vi "00_MOD_Instrument_IO.vi"(8 "error in":errorcluster, 11 "Main Config File Refnum":T2) -> (0 "error out":errorcluster)   [LabVIEW 2018]
doc: "Instrument IO Module main VI. This is the critical Timed loop of the NGTS system. \n\nIt configures DAQmx tasks and channels for PXI, SCXI, and FieldPoint banks for cFP (and future other) instrument buses/cards/modules/banks. The configurations are loaded from tab delimited text files that contain the Tags, Addresses, scaling, polarity, IO type, and other physical IO based Tags. These files are normally located in the \\Config_Files subdirectory. Data IO. Other than an initial channel location .iak file for cFP, all Tags are defined programmatically, without NI-MAX.\n\nIt runs the IO tasks at a nominal 100 mS loop rate. This is adjustable. Data is sent to/from other parts of the system using a Smart VIGlobal, or optionally simple VIGlobals, or RT FIFOs.\n\n2007_11 Mike Ashe\nmichael.ashe@imaginatics.net\nCell: 860-961-0876"
uses:
  <vilib>/Platform/TimedLoop/XDataNode/wakeup.ctl
  <vilib>/Platform/TimedLoop/XDataNode/XDNodeRunTimeDep.lvlib
  <vilib>/Platform/TimedLoop/XDataNode/nitl_modes.ctl
  <vilib>/Platform/TimedLoop/XDataNode/timing_clust.ctl
  <vilib>/Platform/TimedLoop/XDataNode/XDataNode.xnode
  <vilib>/Utility/config.llb/NI_LVConfig.lvlib
  Common/Controls/ENUM Get-Load Action.ctl
  <resource>/objmgr/daqmx.rc
  <vilib>/Utility/config.llb/Read Key (String).vi
  <vilib>/Utility/config.llb/Config Data RefNum.ctl
panel:
  out "x-y":u32
  in  "stop":bool
  out "Period":i64
  out "appended array":dbl[](array[numeric])
  out "error IO":errorcluster
  in  "Error Action":T1(radio)
  in  "Wait On Error?":bool
  in  "Error Wait(mS)":i32=1000
  out "AO Values":dbl[](array[numeric])
  out "Main Loop Period":cluster{i64, "Iteration Duration":i64}(graph)
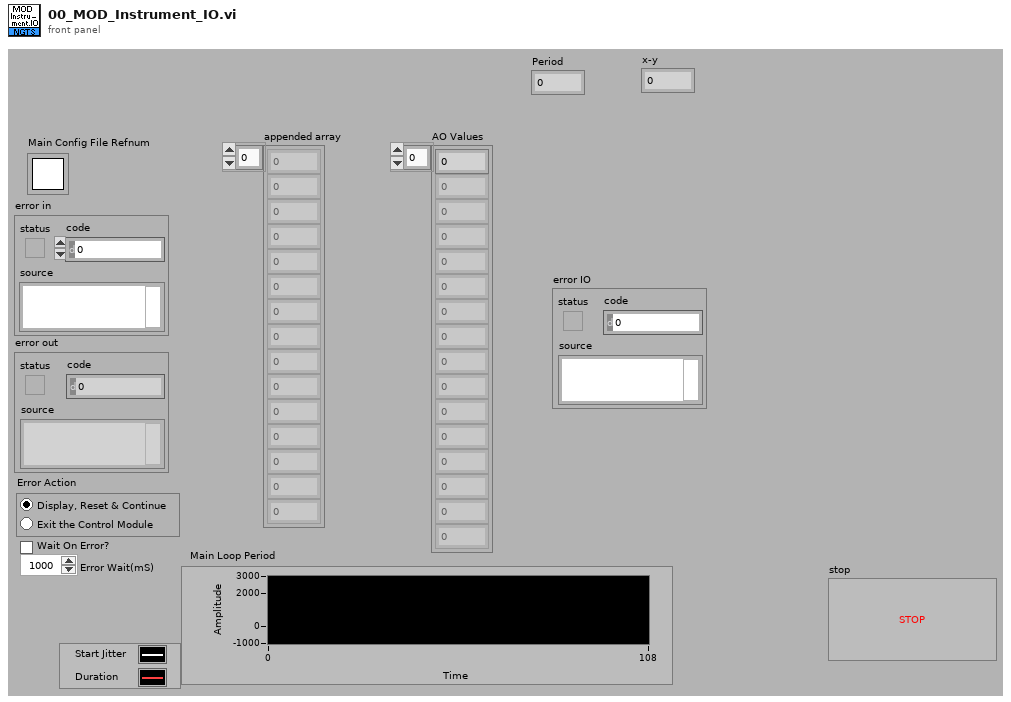
[diagram p1: front panel]
types:
  T1 = enum32{"Display, Reset & Continue", "Exit the Control Module"}
  T2 = typedef "NI_LVConfig.lvlib/Config Data RefNum.ctl" = refnum<k1>
  T3 = typedef "Instrument_IO Shift Variables.ctl" = cluster{"error":errorcluster, "AI_Tasks_State":T4, "AO_Tasks_State":T4, "RUN_PMT_AI":bool, "RUN_PMT_AO":bool, "RUN_PMT_DI":bool, "WDT Time Stamp 1":timestamp, "WDT Time Stamp 2":timestamp, "RT_TO":i32, "WDT_TO":dbl, "AO Tasks":refnum<k21>[], "DI Tasks":refnum<k21>[], "Tag Set Directory":path, "LogPath":path, "DI_Tasks_State":T4, "DO Tasks":refnum<k21>[], "RUN_PMT_DO":bool, "DO_Tasks_State":T4, "LogErrors?":bool, "System Type":string, "AI Sample Rate":dbl, "Timed Loop Rate":dbl, "AI Averaging On":bool, "Agilent Visa Resource":refnum<visa-resource-name>, "FEM Visa Resource":refnum<visa-resource-name>, "AI Tasks":refnum<k21>}
  T4 = typedef "MM_Module_Action.ctl" = enum16{"Idle", "Start", "Run", "Exit"}
  T5 = typedef "XDNodeRunTimeDep.lvlib/timing_clust.ctl" = cluster{"Expected End [f-1]":u64, "Actual End [f-1]":u64, "Finished Late? [f-1]":bool, "Expected End [i-1]":u64, "Actual End [i-1]":u64, "Finished Late? [i-1]":bool, "Expected Start [i]":u64, "Actual Start [i]":u64, "Expected Start [f]":u64, "Actual Start [f]":u64, "Source Name":string, "Structure Name":string, "Period":i64, "Deadline":i64, "Offset":i64, "Start":i64, "Priority":i32, "Timeout":i32, "Mode":T6, "Wakeup Reason":T7, "Error":errorcluster, "Source Type":string, "Secondary Source Type":string, "Global End Time":u64, "Global Start Time":u64, "Frame Duration":u64, "Iteration Duration":u64, "Assigned CPU":i32, "I/O Scan Engine Mode":u32}
  T6 = typedef "XDNodeRunTimeDep.lvlib/nitl_modes.ctl" = enum32{"No Change", "Process missed periods, maintain original phase", "Discard missed periods, maintain original phase", "Process missed periods, ignore original phase", "Discard missed periods, ignore original phase"}
  T7 = typedef "XDNodeRunTimeDep.lvlib/wakeup.ctl" = enum32{"Normal", "Aborted", "Asynchronous wakeup", "Timing source error", "Timed loop error", "Timeout"}
  T8 = typedef "ENUM Get-Load Action.ctl" = enum16{"Get", "Load"}
  T9 = enum16{"get data", "set raw data", "Set Ti and SGi and SGH20", "Add New Formula", "Get Formula", "initialize"}
  T10 = cluster{"Flow (raw gpm)":dbl, "Calibrated Flow (gpm)":dbl, "SG (calibrated)":dbl}
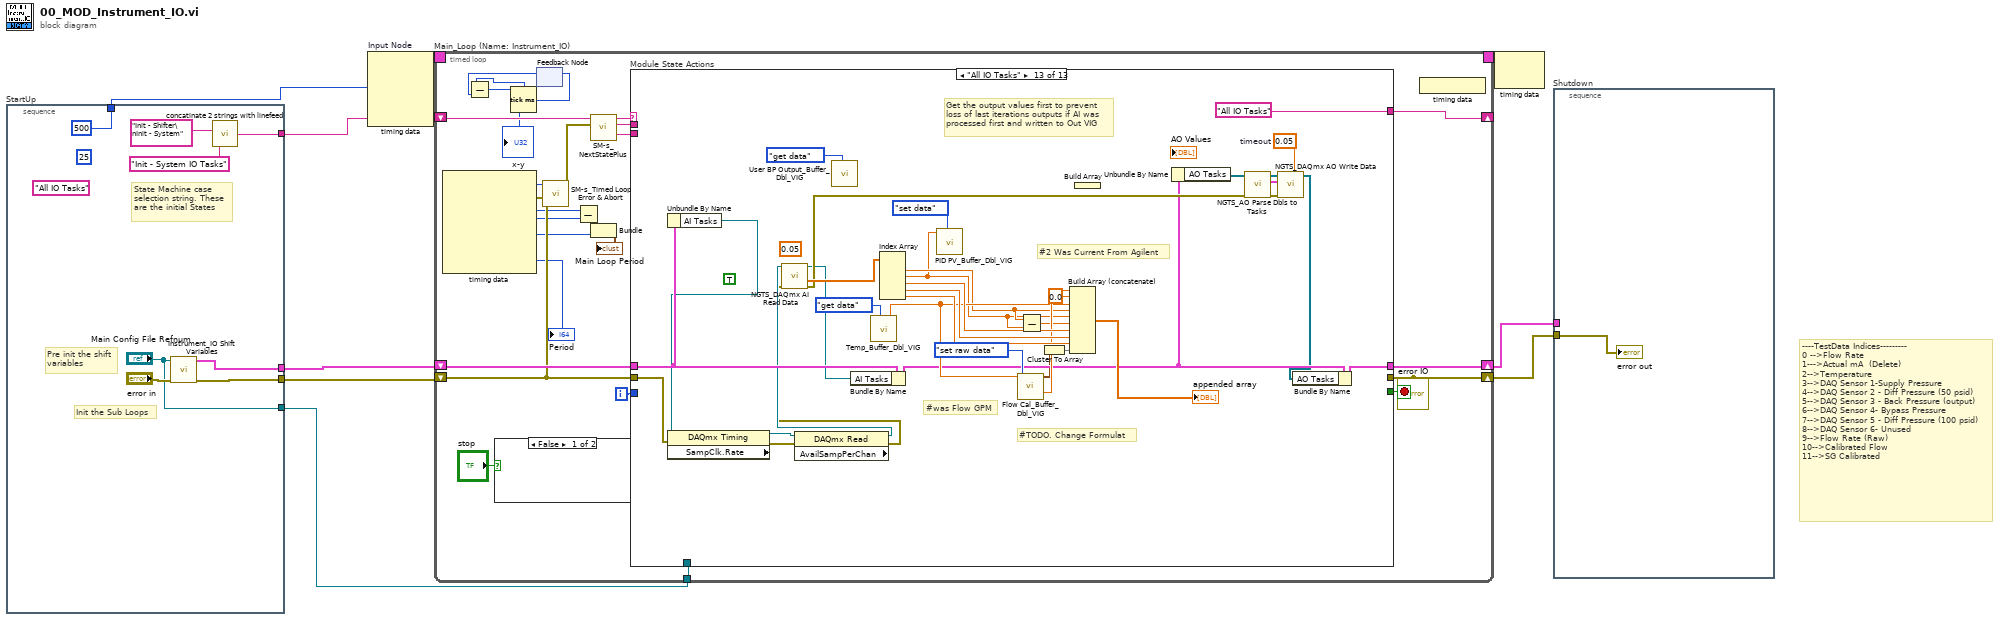
[diagram p0: block diagram]
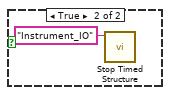
[diagram p2: hidden frame]
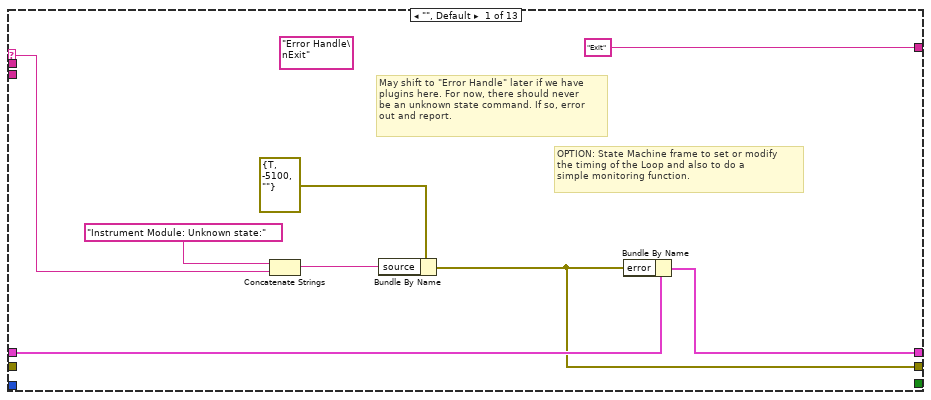
[diagram p3: hidden frame]
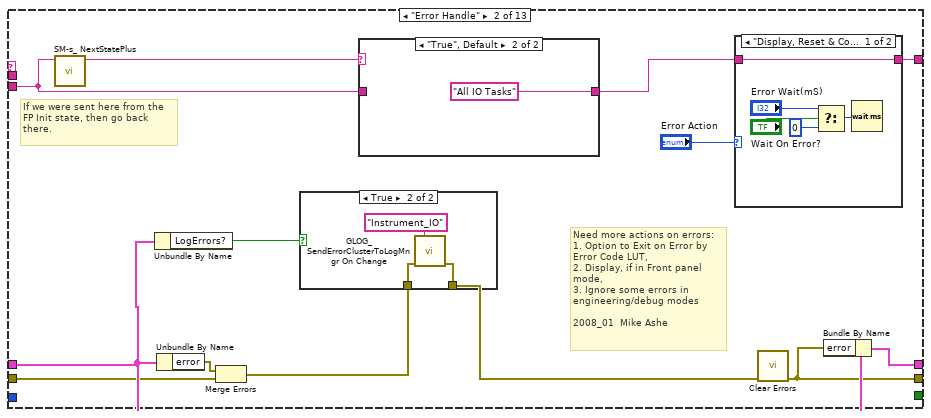
[diagram p4: hidden frame]
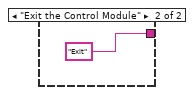
[diagram p6: hidden frame]
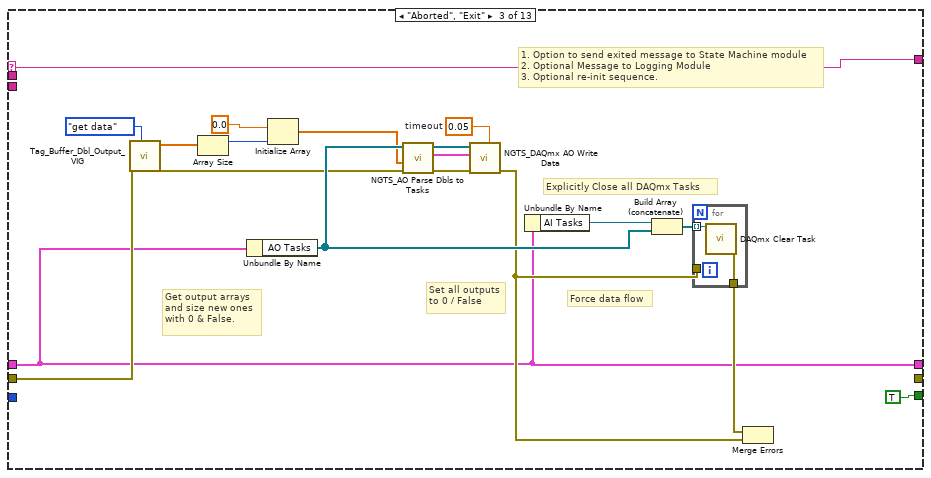
[diagram p8: hidden frame]
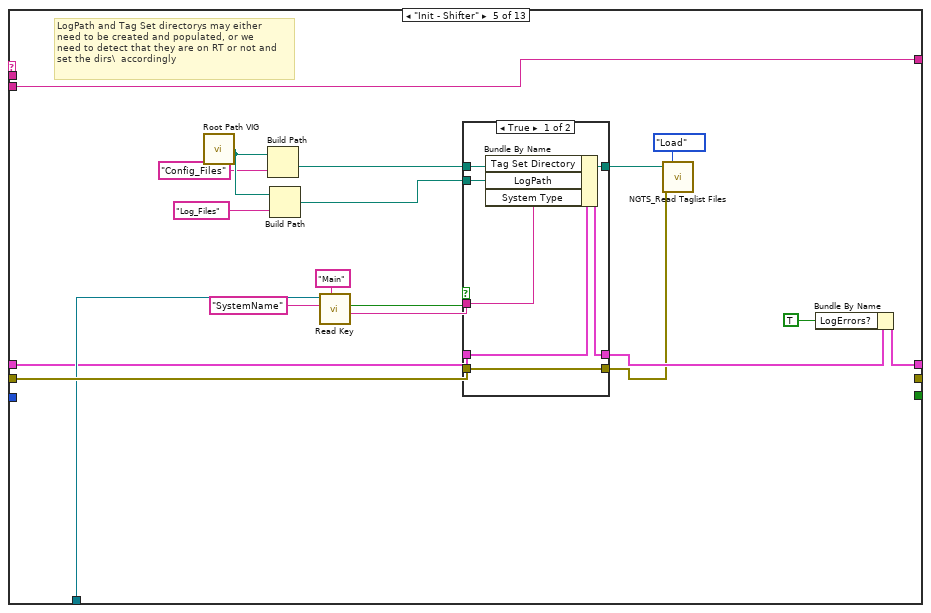
[diagram p10: hidden frame]
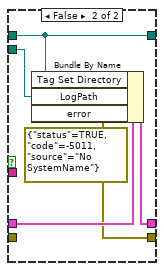
[diagram p11: hidden frame]
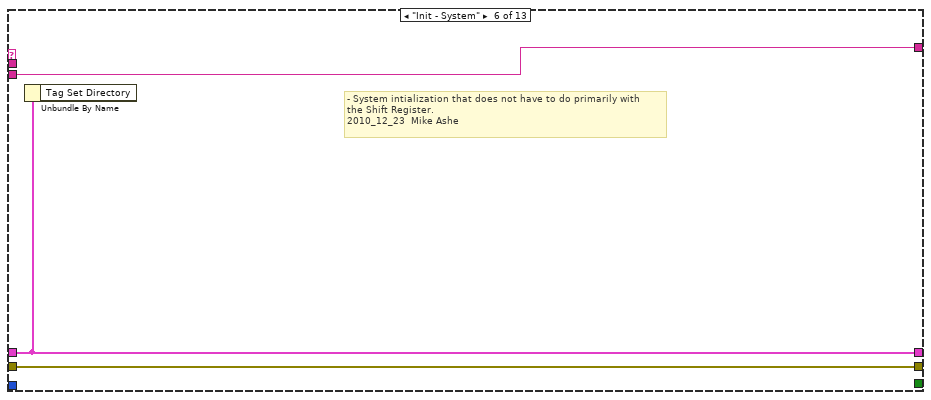
[diagram p12: hidden frame]
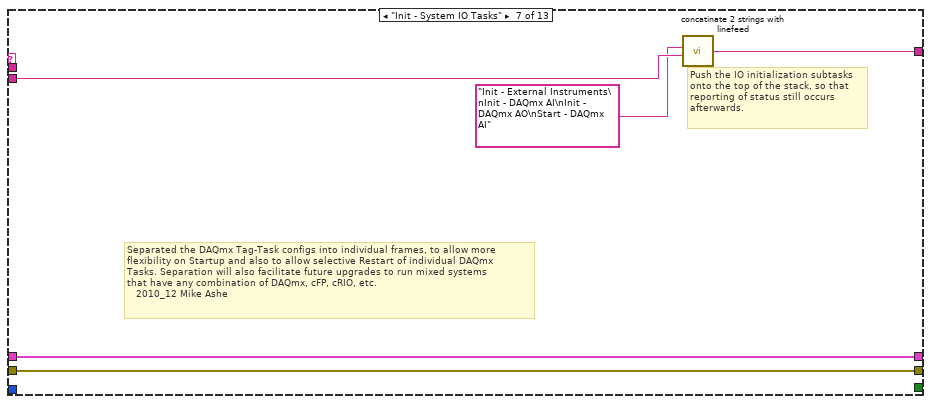
[diagram p13: hidden frame]
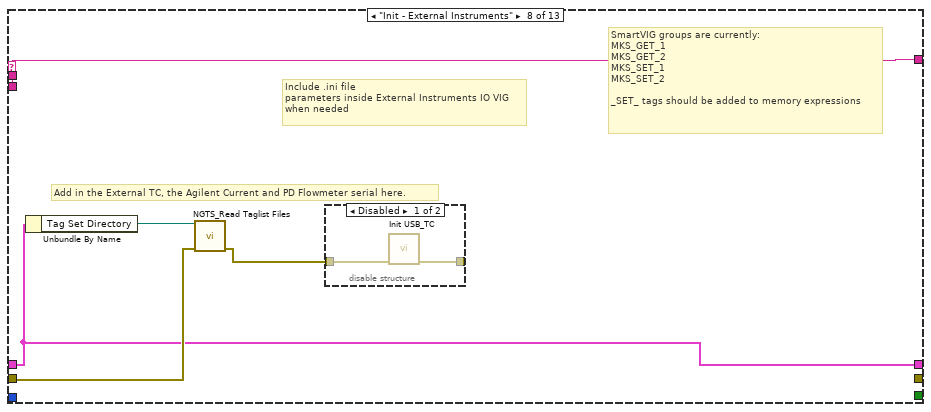
[diagram p14: hidden frame]
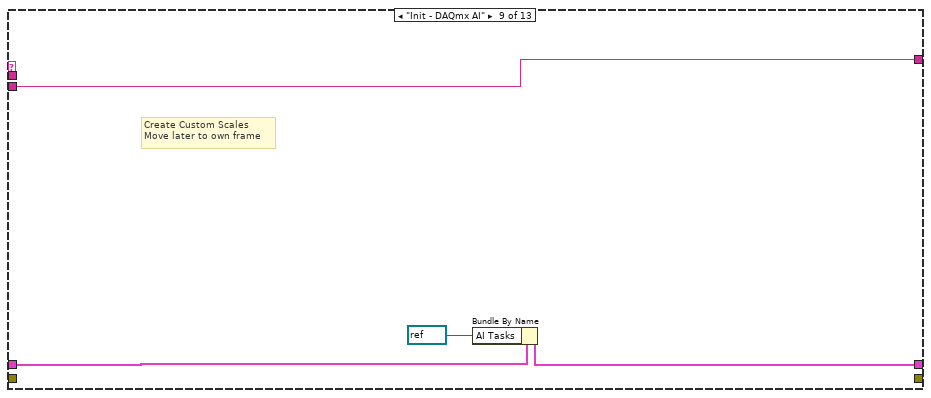
[diagram p16: hidden frame]
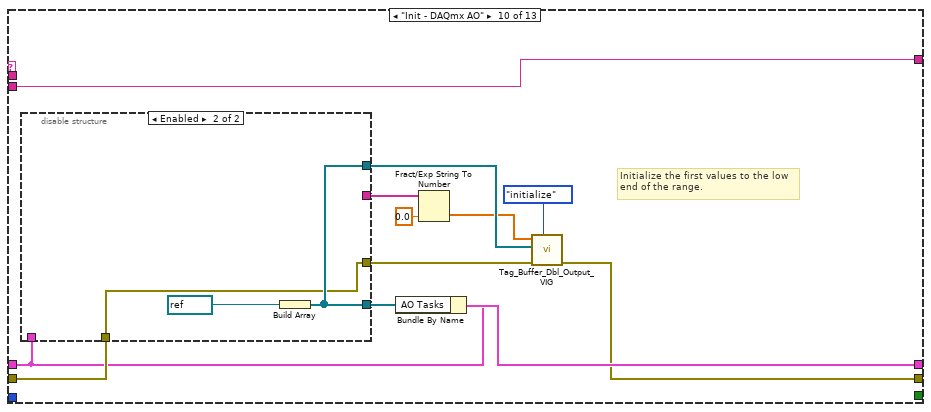
[diagram p17: hidden frame]
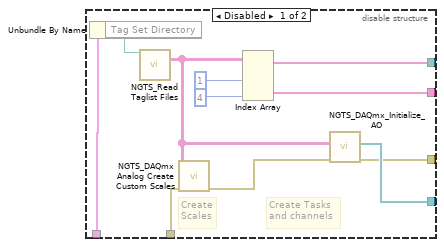
[diagram p18: hidden frame]
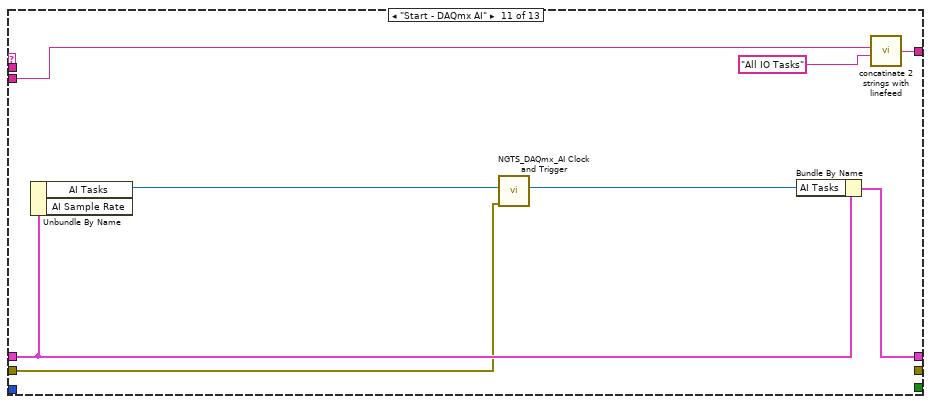
[diagram p19: hidden frame]
diagram:
  # "----TestData Indices---------\n0 -->Flow Rate\n1--->Actual mA  (Delete)\n2-->Temperature\n3-->DAQ Sensor 1-Supply Pressure\n4-->DAQ Sensor 2 - Diff Pressure (50 psid)\n5-->DAQ Sensor 3 - Back Pressure (output)\n6-->DAQ Sensor 4- Bypass Pressure\n7-->DAQ Sensor 5 - Diff Pressure (100 psid)\n8-->DAQ Sensor 6- Unused\n9-->Flow Rate (Raw)\n10-->Calibrated Flow\n11-->SG Calibrated"
  n1 = stacked-sequence "StartUp" {
    tunnel: ["Main Config File Refnum"] -> w1
    tunnel: [w13] -> w7
    tunnel: [500] -> w2
    tunnel: [w15] -> w5
    tunnel: [w12] -> w4
    frame #0 {
      (unwired) "All IO Tasks"
      (unwired) 25
      # "State Machine case \nselection string. These\nare the initial States"
      # "Pre init the shift\nvariables"
      # "Init the Sub Loops"
      n2 = call "Instrument_IO Shift Variables.vi"("error in"="error in", "Main Config File Refnum"="Main Config File Refnum") -> ("error out"=w13:errorcluster, "VARS Instrument_IO"=w12:T3)  [unwired: 8 in]
      n3 = call "concatinate 2 strings with linefeed.vi"("String 2"="Init - System IO Tasks", "String 1"="Init - Shifter\nInit - System") -> ("Concatinated OUT"=w15:string)  [unwired: 6 in]
    }
  }
  n4 = node-c288 "Input Node"(w2) -> (w9:T5)  [unwired: 3 in]
  n5 = timed-loop "Main_Loop (Name: Instrument_IO)" {
    tunnel: w1 -> [w41]
    shift-right: [w23] -> w6
    shift-left: w7 -> [w31]
    shift-right: [w24] -> w3
    shift-left: w4 -> [w40]
    timing: w9 -> [_]
    timing-out: [_] -> w8
    shift-right: [w25] -> _
    shift-left: w5 -> [w38]
    i -> [w42]
    stop <- w39 stop-if-true
    n6 = node-c288() -> (w34:T7, w32:errorcluster, w30:i64, w29:i64, w28:i64, →"Period":i64)  [unwired: 1 in, 1 out]
    n7 = case shown="False" "stop" {
      frame False {
      }
      frame True {
        n8 = call <vilib>:"Stop Timed Structure.vi"("name"="Instrument_IO") -> ()  [unwired: 10 in, 1 out]
      }
    }
    n9 = Tick Count (ms)() -> (millisecond timer value=w19:u32)
    n10 = feedback-in #1(w19) -> ()
    n11 = feedback #1() -> (w20:u32)  [unwired: 1 in]
    n12 = Subtract(x=w19, y=w20) -> (x-y=→"x-y":u32)
    n13 = call "SM-s_Timed Loop Error & Abort.vi"("Error - State In"=w31, "Timed Loop Error In"=w32, "Wakeup Reason"=w34) -> ("error out"=w33:errorcluster)  [unwired: 8 in]
    n14 = Subtract(x=w30, y=w29) -> (x-y=w27:i64)
    n15 = call "SM-s_ NextStatePlus.vi"("error?"=w33, "States String"=w38) -> ("Argument"=w36:string, "Current State"=w37:string, "Next States"=w35:string)  [unwired: 7 in]
    n16 = Bundle(w27, "Iteration Duration"=w28) -> (→"Main Loop Period":cluster{i64, "Iteration Duration":i64})  [unwired: 1 in]
    n17 = case "Module State Actions" shown="\"All IO Tasks\"" w37 {
      selector: w37 -> [w56 _ w102 _ _ _ _ _ _ _ _ _ _]
      tunnel: w42 -> [_ _ _ _ _ _ _ _ _ _ _ _ _]
      tunnel: w41 -> [_ _ _ _ w121 _ _ _ _ _ _ _ _]
      tunnel: w31 -> [_ w63 w86 w106 w122 w140 w144 w150 _ w167 w188 w193 w198]
      tunnel: [w52 w68 _ w106 _ w140 w144 _ _ w162 _ w193 _] -> w23
      tunnel: w40 -> [w58 w71 w85 w107 w110 w139 w146 w147 w156 w164 w192 w194 w225]
      tunnel: [w57 w72 w85 w107 w120 w139 w146 w147 w157 w169 w191 w194 w201] -> w24
      tunnel: [_ _ TRUE _ _ _ _ _ _ _ _ _ _] -> w39
      tunnel: w35 -> [_ w61 _ w108 w127 w141 w143 w151 w158 w170 w187 w195 _]
      tunnel: ["Exit" ("remaining states") w65 w102 w108 w127 w141 w145 w151 w158 w170 w186 w195 "All IO Tasks"] -> w25
      tunnel: w36 -> [_ _ _ _ _ _ _ _ _ _ _ _ _]
      frame "", Default {
        (unwired) "Error Handle\nExit" ("remaining states")
        # "OPTION: State Machine frame to set or modify\nthe timing of the Loop and also to do a\nsimple monitoring function."
        # "May shift to \"Error Handle\" later if we have\nplugins here. For now, there should never\nbe an unknown state command. If so, error\nout and report."
        n18 = Concatenate Strings("Instrument Module: Unknown state:" ("source"), w56) -> (w54:string)
        n19 = Bundle By Name(cluster=errorcluster {"status"=TRUE, "code"=-5100, "source"=""} ("error"), "source"=w54) -> (w52:errorcluster)
        n20 = Bundle By Name(cluster=w58, "error"=w52) -> (w57:T3)
      }
      frame "Error Handle" {
        # "If we were sent here from the\nFP Init state, then go back\nthere."
        # "Need more actions on errors:  \n1. Option to Exit on Error by Error Code LUT,\n2. Display, if in Front panel mode,\n3. Ignore some errors in engineering/debug modes\n\n2008_01  Mike Ashe"
        n21 = call "SM-s_ NextStatePlus.vi"("States String"=w61) -> ("Current State"=w62:string)  [unwired: 8 in, 2 out]
        n22 = Unbundle By Name(w71) -> ("LogErrors?"=w70:bool)
        n23 = Unbundle By Name(w71) -> ("error"=w67:errorcluster)
        n24 = Merge Errors(w67, w63) -> (w60:errorcluster)
        n25 = case shown="True" w70 {
          tunnel: w60 -> [w81 w83]
          tunnel: [w81 w82] -> w69
          frame False {
          }
          frame True {
            n26 = call "GLOG_SendErrorClusterToLogMngr On Change.vi"("System"="Instrument_IO", "error in"=w83) -> ("error out"=w82:errorcluster)  [unwired: 13 in]
          }
        }
        n27 = case shown="\"True\", Default" w62 {
          tunnel: [w73 "All IO Tasks"] -> w66
          tunnel: w61 -> [w73 _]
          frame "Init - FieldPoint ALL" {
          }
          frame "True", Default {
          }
        }
        n28 = case shown="\"Display, Reset & Continue\", Default" "Error Action" {
          tunnel: w66 -> [w75 _]
          tunnel: [w75 "Exit" ("Next States")] -> w65
          frame "Display, Reset & Continue", Default {
            n29 = Select(t="Error Wait(mS)", s="Wait On Error?", f=0) -> (s? t:f=w79:i32)
            n30 = Wait (ms)(milliseconds to wait=w79) -> ()  [unwired: 1 out]
          }
          frame "Exit the Control Module" {
          }
        }
        n31 = call <vilib>:"Clear Errors.vi"("error in (no error)"=w69) -> ("error out"=w68:errorcluster)  [unwired: 5 in, 1 out]
        n32 = Bundle By Name(cluster=w71, "error"=w68) -> (w72:T3)
      }
      frame "Aborted", "Exit" {
        w99 = 0.05  # timeout
        # "Set all outputs\nto 0 / False"
        # "Get output arrays\nand size new ones\nwith 0 & False."
        # "Force data flow"
        # "Explicitly Close all DAQmx Tasks"
        # "1. Option to send exited message to State Machine module\n2. Optional Message to Logging Module\n3. Optional re-init sequence."
        n33 = call "Tag_Buffer_Dbl_Output_VIG.vi"("Operation"=enum16{"get data", "set data", "initialize"}."get data", "error in"=w86) -> ("error out"=w88:errorcluster, "tag_data_out"=w87:dbl[])  [unwired: 7 in, 1 out]
        n34 = Array Size(array=w87) -> (size(s)=w92:i32)
        n35 = Unbundle By Name(w85) -> ("AO Tasks"=w95:refnum<k21>[])
        n36 = Initialize Array(0.0, w92) -> (w93:dbl[])
        n37 = call "NGTS_AO Parse Dbls to Tasks.vi"("error in"=w88, "AO Commands"=w93, "AO Tasks In"=w95) -> ("error out"=w96:errorcluster, "Array"=w97:cluster{"AO Commands":dbl[]}[], "AO Tasks Out"=w98:refnum<k21>[])  [unwired: 6 in]
        n38 = call "NGTS_DAQmx AO Write Data.vi"("timeout"=w99, "error  in"=w96, "AO Data for Tasks"=w97, "AO Tasks In"=w98) -> ("error out"=w90:errorcluster)  [unwired: 6 in, 1 out]
        n39 = Unbundle By Name(w85) -> ("AI Tasks"=w101:refnum<k21>)
        n40 = Build Array (concatenate)(w101, w95) -> (w100:refnum<k21>[])
        n41 = for {
          tunnel: w100 -> [w105] mode=indexing
          tunnel: [w104] -> w94
          tunnel: w90 -> [_]
          n42 = call <vilib>:"DAQmx Clear Task.vi"("task in"=w105) -> ("error out"=w104:errorcluster)  [unwired: 14 in]
        }
        n43 = Merge Errors(w94, w90) -> ()  [unwired: 1 out]
      }
      frame "----- Initialization Actions -----" {
        # "This frame should never actually run. It is used to delineate the\ngroupings in the State machine"
      }
      frame "Init - Shifter" {
        # "LogPath and Tag Set directorys may either\nneed to be created and populated, or we\nneed to detect that they are on RT or not and\nset the dirs\\  accordingly"
        n44 = call "Root Path VIG.vi"() -> ("Root VI's Path"=w114:path)  [unwired: 1 in]
        n45 = Build Path(base path=w114, name or relative path="Config_Files") -> (appended path=w109:path)
        n46 = Build Path(base path=w114, name or relative path="Log_Files") -> (appended path=w111:path)
        n47 = call-poly <vilib>:"Read Key.vi"("section"="Main", "key"="SystemName", "refnum"=w121) -> ("value"=w124:string, "found?"=w123:bool)  [unwired: 5 in, 2 out]
        n48 = case shown="True" w123 {
          tunnel: [w133 w138] -> w119
          tunnel: w109 -> [w128 w134]
          tunnel: w110 -> [w132 w137]
          tunnel: w111 -> [w131 w136]
          tunnel: w124 -> [w130 _]
          tunnel: w122 -> [w129 _]
          tunnel: [w129 w135] -> w115
          tunnel: [w128 w134] -> w117
          frame True {
            n49 = Bundle By Name(cluster=w132, "Tag Set Directory"=w128, "LogPath"=w131, "System Type"=w130) -> (w133:T3)
          }
          frame False {
            w135 = errorcluster {"status"=TRUE, "code"=-5011, "source"="No SystemName"} ("error out")
            n50 = Bundle By Name(cluster=w137, "Tag Set Directory"=w134, "LogPath"=w136, "error"=w135) -> (w138:T3)
          }
        }
        n51 = call "NGTS_Read Taglist Files.vi"("Tag Set Directory"=w117, "Get-Load Action"=ENUM_Get-Load_Action."Load", "error in"=w115) -> ()  [unwired: 6 in, 7 out]
        n52 = Bundle By Name(cluster=w119, "LogErrors?"=TRUE) -> (w120:T3)
      }
      frame "Init - System" {
        # "- System intialization that does not have to do primarily with\nthe Shift Register.\n2010_12_23  Mike Ashe"
        n53 = Unbundle By Name(w139) -> ()  [unwired: 1 out]
      }
      frame "Init - System IO Tasks" {
        # "Push the IO initialization subtasks\nonto the top of the stack, so that\nreporting of status still occurs \nafterwards."
        # "Separated the DAQmx Tag-Task configs into individual frames, to allow more\nflexibility on Startup and also to allow selective Restart of individual DAQmx\nTasks. Separation will also facilitate future upgrades to run mixed systems\nthat have any combination of DAQmx, cFP, cRIO, etc.\n   2010_12 Mike Ashe"
        n54 = call "concatinate 2 strings with linefeed.vi"("String 2"=w143, "String 1"="Init - External Instruments\nInit - DAQmx AI\nInit - DAQmx AO\nStart - DAQmx AI") -> ("Concatinated OUT"=w145:string)  [unwired: 6 in]
      }
      frame "Init - External Instruments" {
        # "Add in the External TC, the Agilent Current and PD Flowmeter serial here."
        # "SmartVIG groups are currently:\nMKS_GET_1\nMKS_GET_2\nMKS_SET_1\nMKS_SET_2\n\n_SET_ tags should be added to memory expressions"
        # "Include .ini file\nparameters inside External Instruments IO VIG\nwhen needed"
        n55 = Unbundle By Name(w147) -> ("Tag Set Directory"=w149:path)
        n56 = call "NGTS_Read Taglist Files.vi"("Tag Set Directory"=w149, "error in"=w150) -> ("error out"=w148:errorcluster)  [unwired: 7 in, 6 out]
        n57 = disable-structure shown="Disabled" {
          disable-tunnel: w148 -> [w153 w154]
          disable-tunnel: [w152 w154] -> _
          frame Disabled {
            n58 = call "Init USB_TC.vi"("error in"=w153) -> ("error out"=w152:errorcluster)  [unwired: 9 in, 1 out]
          }
          frame Enabled {
          }
        }
      }
      frame "Init - DAQmx AI" {
        # "Create Custom Scales\nMove later to own frame"
        n59 = Bundle By Name(cluster=w156, "AI Tasks"=refnum<k21> "AI" ("task out")) -> (w157:T3)
      }
      frame "Init - DAQmx AO" {
        # "Initialize the first values to the low\nend of the range."
        n60 = disable-structure shown="Enabled" {
          disable-tunnel: [w181 w183] -> w168
          disable-tunnel: w167 -> [w179 w182]
          disable-tunnel: [w174 _] -> w166
          disable-tunnel: w164 -> [w173 _]
          disable-tunnel: [w172 w182] -> w163
          disable-tunnel: [w171 w183] -> w161
          frame Disabled {
            # "Create Tasks\nand channels"
            # "Create\nScales"
            n61 = Unbundle By Name(w173) -> ("Tag Set Directory"=w180:path)
            n62 = call "NGTS_Read Taglist Files.vi"("Tag Set Directory"=w180) -> ("AO Channels Properties Table"=w176:string[][])  [unwired: 8 in, 6 out]
            n63 = call "NGTS_DAQmx Analog Create Custom Scales.vi"("error in"=w179, "Channels Properties Table"=w176) -> ("error out"=w178:errorcluster)  [unwired: 7 in, 2 out]
            n64 = Index Array(array=w176, index (col) #1=1 ("disabled index (col)"), index (col) #2=4 ("disabled index (col)")) -> (element #1=w171:string[], element #2=w174:string[])  [unwired: 2 in]
            n65 = call "NGTS_DAQmx_Initialize_AO.vi"("error in"=w178, "Channels Properties Table"=w176) -> ("error out"=w172:errorcluster, "AO Task Array Out"=w181:refnum<k21>[])  [unwired: 8 in]
          }
          frame Enabled {
            n66 = Build Array(refnum<k21> "AO" ("task out")) -> (w183:refnum<k21>[])
          }
        }
        n67 = Bundle By Name(cluster=w164, "AO Tasks"=w168) -> (w169:T3)
        n68 = Fract/Exp String To Number(string=w166, default (0 dbl)=0.0 ("default (0 DBL)")) -> (number=w160:dbl[])  [unwired: 2 in, 1 out]
        n69 = call "Tag_Buffer_Dbl_Output_VIG.vi"("Operation"=enum16{"get data", "set data", "initialize"}."initialize", "error in"=w163, "tag_names_in"=w161, "tag_data_in"=w160) -> ("error out"=w162:errorcluster)  [unwired: 5 in, 2 out]
      }
      frame "Start - DAQmx AI" {
        n70 = Unbundle By Name(w192) -> ("AI Tasks"=w190:refnum<k21>)  [unwired: 1 out]
        n71 = call "NGTS_DAQmx_AI Clock and Trigger.vi"("error in"=w188, "AI Tasks In"=w190) -> ("AI Tasks Out"=w189:refnum<k21>)  [unwired: 8 in, 1 out]
        n72 = Bundle By Name(cluster=w192, "AI Tasks"=w189) -> (w191:T3)
        n73 = call "concatinate 2 strings with linefeed.vi"("String 2"="All IO Tasks", "String 1"=w187) -> ("Concatinated OUT"=w186:string)  [unwired: 6 in]
      }
      frame "----- Instrument Actions -----" {
        # "This frame should never actually run. It is used to delineate the\ngroupings in the State machine"
      }
      frame "All IO Tasks" {
        (unwired) TRUE ("AI Averaging On")
        w230 = 0.05  # timeout
        (unwired) 0.05 ("timeout")
        # "#was Flow GPM"
        # "#2 Was Current From Agilent"
        # "#TODO. Change Formulat"
        # "Get the output values first to prevent\nloss of last iterations outputs if AI was\nprocessed first and written to Out VIG"
        n74 = Unbundle By Name(w225) -> ("AI Tasks"=w205:refnum<k21>)
        n75 = property class="DAQmx Timing" props=["SampClk.Rate"](reference=w205, error in=w198) -> (reference out=w206:refnum<k21>, error out=w207:errorcluster)  [unwired: 1 out]
        n76 = property class="DAQmx Read" props=["AvailSampPerChan"](reference=w206, error in=w207) -> (reference out=w204:refnum<k21>, error out=w199:errorcluster)  [unwired: 1 out]
        n77 = call "NGTS_DAQmx AI Read Data.vi"("error  in"=w199, "AI Tasks In"=w204) -> ("error out"=w222:errorcluster, "Raw 1D Data out"=w223:dbl[], "AI Tasks Out"=w202:refnum<k21>)  [unwired: 7 in]
        n78 = call "User BP Output_Buffer_Dbl_VIG.vi"("Operation"=enum16{"get data", "set data", "initialize"}."get data") -> ()  [unwired: 9 in, 2 out]
        n79 = Bundle By Name(cluster=w225, "AI Tasks"=w202) -> (w203:T3)
        n80 = call "Temp_Buffer_Dbl_VIG.vi"("Operation"=enum16{"get data", "set data", "initialize"}."get data") -> ("Numeric"=w213:dbl)  [unwired: 9 in, 1 out]
        n81 = Index Array(array=w223) -> (element #1=w210:dbl, element #2=w209:dbl, element #3=w219:dbl, element #4=w218:dbl, element #5=w217:dbl)  [unwired: 5 in]
        n82 = call "PID PV_Buffer_Dbl_VIG.vi"("Operation"=enum16{"get data", "set data", "initialize"}."set data", "Numeric"=w209) -> ()  [unwired: 8 in, 2 out]
        n83 = call "Flow Cal_Buffer_Dbl_VIG.vi"("Fuel Temp"=w213, "Operation"=T9."set raw data") -> ("Addtional Values"=w197:T10, "Calibrated Flow (lb/hr)"=w216:dbl)  [unwired: 10 in, 2 out]
        n84 = Subtract(x=w210, y=w209) -> (x-y=w208:dbl)
        n85 = Cluster To Array(cluster=w197) -> (array=w215:dbl[])
        n86 = Build Array (concatenate)(w216, 0.0 ("element"), w213, w210, w209, w208, w219, w218, w217, w215) -> (→"appended array":dbl[])
        n87 = Build Array() -> ()  [unwired: 1 in, 1 out]
        n88 = Unbundle By Name(w203) -> ("AO Tasks"=w224:refnum<k21>[])
        n89 = call "NGTS_AO Parse Dbls to Tasks.vi"("error in"=w222, "AO Tasks In"=w224) -> ("error out"=w226:errorcluster, "Array"=w227:cluster{"AO Commands":dbl[]}[], "AO Tasks Out"=w228:refnum<k21>[])  [unwired: 7 in]
        n90 = call "NGTS_DAQmx AO Write Data.vi"("timeout"=w230, "error  in"=w226, "AO Data for Tasks"=w227, "AO Tasks In"=w228) -> ("AO Tasks Out"=w200:refnum<k21>[])  [unwired: 6 in, 1 out]
        n91 = Bundle By Name(cluster=w203, "AO Tasks"=w200) -> (w201:T3)
      }
    }
    "error IO" <- w23
    n92 = node-c288() -> ()  [unwired: 1 out]
  }
  n93 = node-c288(w8) -> ()  [unwired: 1 out]
  n94 = stacked-sequence "Shutdown" {
    tunnel: w6 -> [w231]
    tunnel: w3 -> [_]
    frame #0 {
      "error out" <- w231
    }
  }
